vi "Get Tag Types.vi"(3 "Error In":errorcluster, 5 "Database Connection":refnum<k7>) -> (0 "Error Out":errorcluster, 1 "TagTypeNames":string[](array[string]), 2 "TagTypeIds":string[](array[string]))   [LabVIEW 2019]
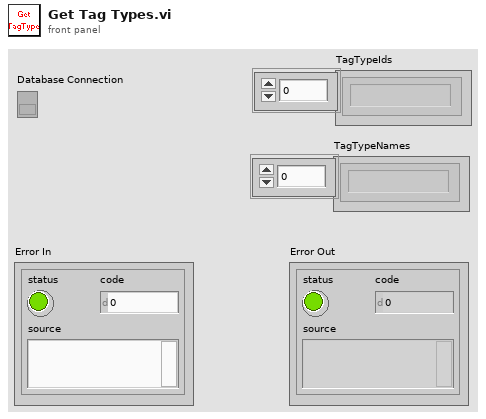
[diagram p1: front panel]
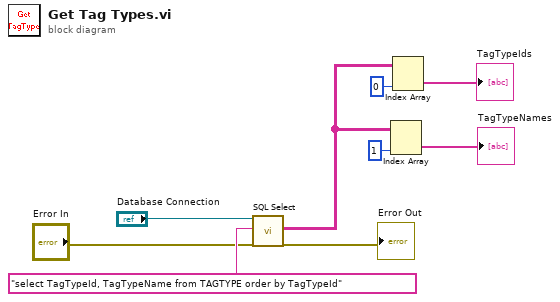
[diagram p0: block diagram]
diagram:
  n1 = call <vilib>:"SQL Select.vi"("Connection In"="Database Connection", "SQL Query"="select TagTypeId, TagTypeName from TAGTYPE order by TagTypeId", "Error in (no error)"="Error In") -> ("Data"=w2:string[][], "Error out"=→"Error Out":errorcluster)  [unwired: 14 in, 1 out]
  n2 = Index Array(array=w2, index (col)=1 ("disabled index (col)")) -> (element=→"TagTypeNames":string[])  [unwired: 1 in]
  n3 = Index Array(array=w2, index (col)=0 ("disabled index (col)")) -> (element=→"TagTypeIds":string[])  [unwired: 1 in]
